vi "Configure Multi Eval Meas Limit Power Dynamics Test Tolerances For Channel BW.vi"(7 "Power Great 3 GHz (0.0)":dbl format="%^.3e", 8 "error in (no error)":errorcluster, 9 "Power Less 3 GHz (0.0)":dbl format="%^.3e", 10 "Instance (1)":T1=1, 11 "VISA resource name":refnum<visa-resource-name>) -> (0 "error out":errorcluster, 3 "VISA resource name out":refnum<visa-resource-name>)   [LabVIEW 2020, in "Rohde&Schwarz CMWXP NR FR1 Measurement.lvlib"]
doc: "Defines test tolerances for power dynamics limits, for channel BW up to 40 MHz.\n\nAttribute:\nRSCMWXPNRFR1M_ATTR_MULTI_EVAL_MEAS_LIMIT_POWER_DYNAMICS_TEST_TOLERANCES_FOR_CHANNEL_BW\n\nRemote-control command:\nCONFigure:NRSub:MEAS<i>:MEValuation:LIMit:PDYNamics:TTOLerance:CBLT"
uses:
  <instrlib>/Rohde&Schwarz CMWXP NR FR1 Measurement/Rohde&Schwarz CMWXP NR FR1 Measurement.lvlib
  <instrlib>/Rohde&Schwarz CMWXP NR FR1 Measurement/Private/_Instance.ctl
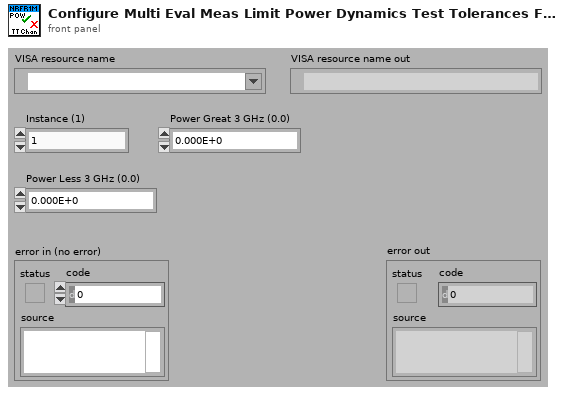
[diagram p1: front panel]
types:
  T1 = typedef "Rohde&Schwarz CMWXP NR FR1 Measurement.lvlib/_Instance.ctl" = i32
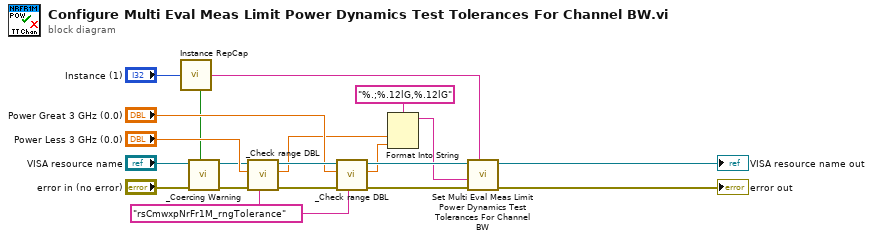
[diagram p0: block diagram]
diagram:
  w10 = "rsCmwxpNrFr1M_rngTolerance" ("Range Table Identifier")
  n1 = call <instrlib>:"Instance RepCap.vi"("Instance In"="Instance (1)") -> ("In Range?"=w1:bool, "RepCap Identifier Out"=w17:string)  [unwired: 1 in]
  n2 = call <instrlib>:"_Coercing Warning.vi"("In Range?"=w1, "error in (no error)"="error in (no error)", "VISA resource name"="VISA resource name") -> ("error out"=w3:errorcluster, "VISA resource name out"=w2:refnum<visa-resource-name>)  [unwired: 7 in]
  n3 = call <instrlib>:"_Check range DBL.vi"("Range Table Identifier"=w10, "error in (no error)"=w3, "DBL Value In"="Power Less 3 GHz (0.0)", "VISA resource name"=w2) -> ("error out"=w16:errorcluster, "DBL Value Out"=w8:dbl, "VISA resource name out"=w15:refnum<visa-resource-name>)  [unwired: 5 in]
  n4 = call <instrlib>:"_Check range DBL.vi"("Range Table Identifier"=w10, "error in (no error)"=w16, "DBL Value In"="Power Great 3 GHz (0.0)", "VISA resource name"=w15) -> ("error out"=w14:errorcluster, "DBL Value Out"=w7:dbl, "VISA resource name out"=w13:refnum<visa-resource-name>)  [unwired: 5 in]
  n5 = Format Into String(format string="%.;%.12lG,%.12lG", w8, w7) -> (resulting string=w6:string)  [unwired: 2 in, 1 out]
  n6 = call "Set Multi Eval Meas Limit Power Dynamics Test Tolerances For Channel BW"("Repeated Capabilities"=w17, "error in (no error)"=w14, "Multi Eval Meas Limit Power Dynamics Test Tolerances For Channel BW ()"=w6, "instrument handle"=w13) -> ("error out"=→"error out":errorcluster, "instrument handle out"=→"VISA resource name out":refnum<visa-resource-name>)  [unwired: 6 in]
